vi "Configure Relay.vi"(0 "VISA resource name":refnum<visa-resource-name>, 5 "Relay (1:Relay 1)":u16(ring)=1 items=["Relay 1"=1, "Relay 2"=2], 7 "Relay Mode (0:Off)":u16(ring) items=["Manual Off", "Manual On", "Alarms"], 9 "Input Alarm (0:Input A)":u16(ring) items=["Input A", "Input B", "Input C", "Input D"], 11 "error in (no error)":errorcluster, 12 "Alarm Type (0:Low Alarm)":u16(ring) items=["Low Alarm", "High Alarm", "Both Alarms"]) -> (4 "VISA resource name out":refnum<visa-resource-name>, 15 "error out":errorcluster)   [LabVIEW 2017, in "Lake Shore 336.lvlib"]
doc: "This VI configures the Model 336 relays. The Model 336 has two relays that may be operated manually or tied to input alarms."
uses:
  Lake Shore 336.lvlib
  Instance           1 23Saved   Configure Relay .vi
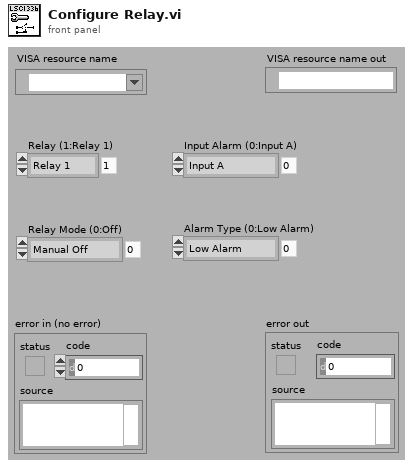
[diagram p1: front panel]
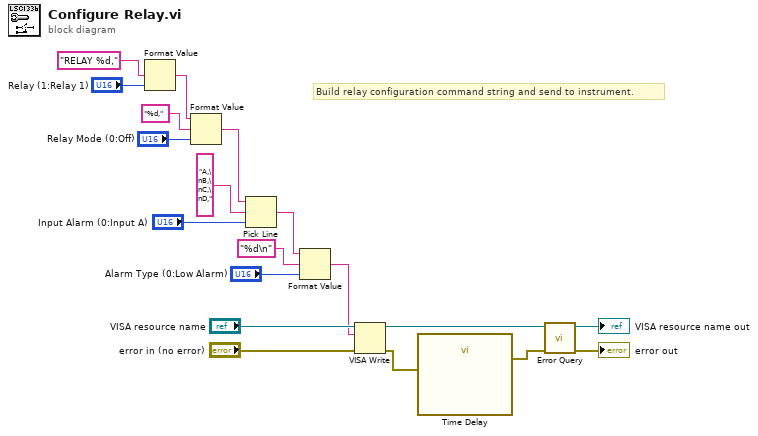
[diagram p0: block diagram]
diagram:
  # "Build relay configuration command string and send to instrument."
  n1 = Format Value(format string="RELAY %d,", value (0)="Relay (1:Relay 1)") -> (output string=w9:string)  [unwired: 1 in]
  n2 = Format Value(string ("")=w9, format string="%d,", value (0)="Relay Mode (0:Off)") -> (output string=w5:string)
  n3 = Pick Line(string ("")=w5, multi-line string="A,\nB,\nC,\nD,", line index="Input Alarm (0:Input A)") -> (output string=w3:string)
  n4 = Format Value(string ("")=w3, format string="%d\n", value (0)="Alarm Type (0:Low Alarm)") -> (output string=w1:string)
  n5 = VISA Write(VISA resource name="VISA resource name", write buffer=w1, error in (no error)="error in (no error)") -> (VISA resource name out=w17:refnum<visa-resource-name>, error out=w13:errorcluster)  [unwired: 1 out]
  n6 = call "Time Delay"("error in (no error)"=w13) -> ("error out"=w12:errorcluster)  [unwired: 10 in]
  n7 = call "Error Query.vi"("error in (no error)"=w12, "VISA resource name"=w17) -> ("error out"=→"error out":errorcluster, "VISA resource name out"=→"VISA resource name out":refnum<visa-resource-name>)  [unwired: 7 in, 1 out]
